vi "Go To Position.vi"(8 "error in (no error)":errorcluster, 10 "Desired Position":dbl, 11 "DAQ Digital Code Scan in":refnum<class "DAQ Digital Code Scan.lvclass">) -> (0 "error out":errorcluster, 2 "Current Position":dbl, 3 "DAQ Digital Code Scan out":refnum<class "DAQ Digital Code Scan.lvclass">)   [LabVIEW 2012, in "DAQ Digital Code Scan.lvclass"]
uses:
  DAQ Digital Code Scan.lvclass
  DAQ Digital Code Scan.lvclass/DAQ Digital Code Scan.ctl
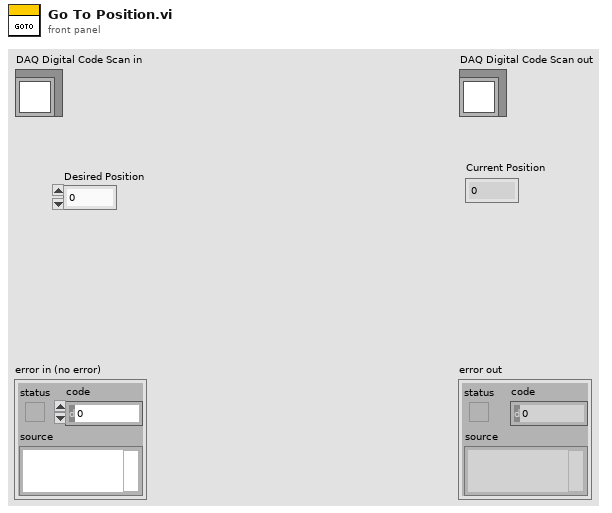
[diagram p1: front panel]
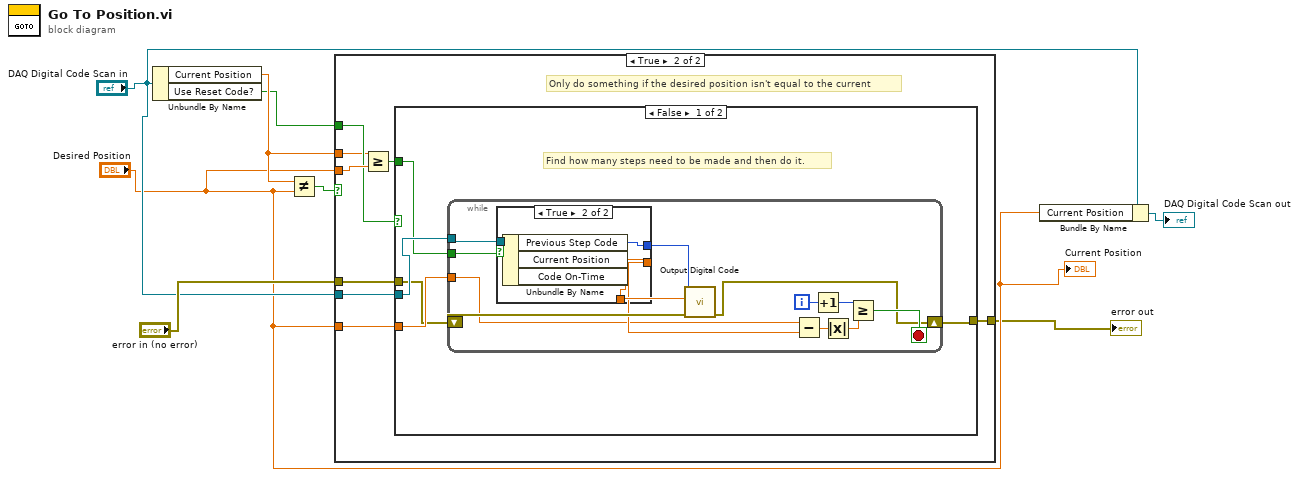
[diagram p0: block diagram]
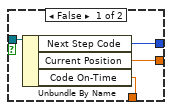
[diagram p3: hidden frame]
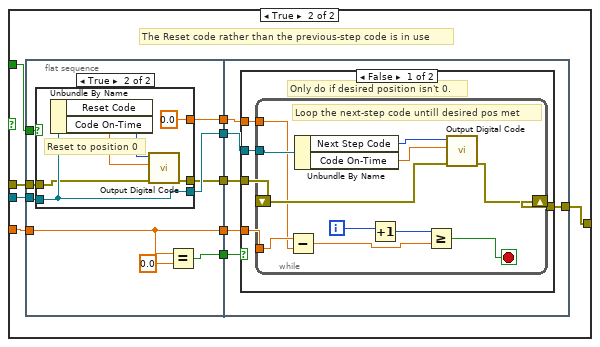
[diagram p4: hidden frame]
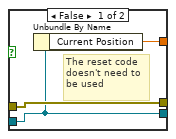
[diagram p5: hidden frame]
diagram:
  n1 = Unbundle By Name("DAQ Digital Code Scan in") -> ("Current Position"=w7:dbl, "Use Reset Code?"=w6:bool)
  n2 = Not Equal?(x=w7, y="Desired Position") -> (x != y?=w8:bool)
  n3 = case shown="True" w8 {
    tunnel: w7 -> [_ w10]
    tunnel: "Desired Position" -> [_ w17]
    tunnel: w6 -> [_ w15]
    tunnel: "DAQ Digital Code Scan in" -> [_ w14]
    tunnel: "error in (no error)" -> [w9 w13]
    tunnel: "Desired Position" -> [_ w12]
    tunnel: [w9 w11] -> w1
    frame False {
    }
    frame True {
      # "Only do something if the desired position isn't equal to the current"
      n4 = Greater Or Equal?(x=w10, y=w17) -> (x >= y?=w16:bool)
      n5 = case shown="False" w15 {
        tunnel: w16 -> [w19 w53]
        tunnel: w14 -> [w22 w52]
        tunnel: w13 -> [w20 w50]
        tunnel: w12 -> [w21 w48]
        tunnel: [w18 w46] -> w11
        frame False {
          # "Find how many steps need to be made and then do it."
          n6 = while {
            tunnel: w22 -> [w33]
            tunnel: w21 -> [w26]
            shift-right: [w31] -> w18
            shift-left: w20 -> [w32]
            tunnel: w19 -> [w25]
            i -> [w29]
            stop <- w34 stop-if-true
            n7 = case shown="True" w25 {
              tunnel: [w39 w42] -> w35
              tunnel: w33 -> [w38 w43]
              tunnel: [w37 w40] -> w30
              tunnel: [w36 w41] -> w27
              frame False {
                n8 = Unbundle By Name(w38) -> ("Next Step Code"=w39:i8, "Current Position"=w36:dbl, "Code On-Time"=w37:dbl)
              }
              frame True {
                n9 = Unbundle By Name(w43) -> ("Previous Step Code"=w42:i8, "Current Position"=w41:dbl, "Code On-Time"=w40:dbl)
              }
            }
            n10 = call "Output Digital Code.vi"("error in (no error)"=w32, "Pulse Time"=w30, "Input"=w35) -> ("error out"=w31:errorcluster)  [unwired: 6 in]
            n11 = Subtract(x=w26, y=w27) -> (x-y=w23:dbl)
            n12 = Increment(x=w29) -> (x+1=w28:i32)
            n13 = Absolute Value(x=w23) -> (abs(x)=w24:dbl)
            n14 = Greater Or Equal?(x=w28, y=w24) -> (x >= y?=w34:bool)
          }
        }
        frame True {
          # "The Reset code rather than the previous-step code is in use"
          n15 = flat-sequence {
            tunnel: w53 -> [w62]
            tunnel: w52 -> [w61]
            tunnel: [w60] -> w51
            tunnel: w50 -> [w59]
            tunnel: [w58] -> w49
            tunnel: w48 -> [w57]
            tunnel: [w57] -> w47
            tunnel: [w56] -> w45
            tunnel: [w54] -> w44
            tunnel: w51 -> [w77]
            tunnel: w49 -> [w76]
            tunnel: w47 -> [w75]
            tunnel: [w74] -> w46
            tunnel: w45 -> [w73]
            tunnel: w44 -> [w72]
            frame #0 {
              n16 = case shown="True" w62 {
                tunnel: w61 -> [w64 w69]
                tunnel: [w64 w69] -> w60
                tunnel: w59 -> [w65 w68]
                tunnel: [w65 w67] -> w58
                tunnel: [w63 0.0 ("Current Position")] -> w54
                frame False {
                  # "The reset code\ndoesn't need to\nbe used"
                  n17 = Unbundle By Name(w64) -> ("Current Position"=w63:dbl)
                }
                frame True {
                  # "Reset to position 0"
                  n18 = Unbundle By Name(w69) -> ("Reset Code"=w71:i8, "Code On-Time"=w70:dbl)
                  n19 = call "Output Digital Code.vi"("error in (no error)"=w68, "Pulse Time"=w70, "Input"=w71) -> ("error out"=w67:errorcluster)  [unwired: 6 in]
                }
              }
              n20 = Equal?(x=w57, y=0.0) -> (x = y?=w56:bool)
            }
            frame #1 {
              n21 = case shown="False" w73 {
                tunnel: w77 -> [w82 _]
                tunnel: w76 -> [w81 w94]
                tunnel: w75 -> [w80 _]
                tunnel: [w79 w94] -> w74
                tunnel: w72 -> [w78 _]
                frame False {
                  # "Only do if desired position isn't 0."
                  n22 = while {
                    tunnel: w80 -> [w85]
                    shift-right: [w89] -> w79
                    shift-left: w81 -> [w90]
                    tunnel: w82 -> [w86]
                    tunnel: w78 -> [w84]
                    i -> [w87]
                    stop <- w93 stop-if-true
                    # "Loop the next-step code untill desired pos met"
                    n23 = Subtract(x=w85, y=w84) -> (x-y=w83:dbl)
                    n24 = Unbundle By Name(w86) -> ("Next Step Code"=w92:i8, "Code On-Time"=w91:dbl)
                    n25 = Increment(x=w87) -> (x+1=w88:i32)
                    n26 = Greater Or Equal?(x=w88, y=w83) -> (x >= y?=w93:bool)
                    n27 = call "Output Digital Code.vi"("error in (no error)"=w90, "Pulse Time"=w91, "Input"=w92) -> ("error out"=w89:errorcluster)  [unwired: 6 in]
                  }
                }
                frame True {
                  # "Desired position already met"
                }
              }
            }
          }
        }
      }
    }
  }
  "error out" <- w1
  n28 = Bundle By Name(cluster="DAQ Digital Code Scan in", "Current Position"="Desired Position") -> (→"DAQ Digital Code Scan out":refnum<class "DAQ Digital Code Scan.lvclass">)
  "Current Position" <- "Desired Position"
